vi "適應性控制_線上學習_V7(實際控制).vi"() -> ()   [LabVIEW 2010]
uses:
  <vilib>/DAQmx/read.llb/DAQmx Read (Analog 1D Wfm NChan NSamp).vi
  <vilib>/DAQmx/write.llb/DAQmx Write (Analog DBL 1Chan 1Samp).vi
  <vilib>/DAQmx/create/channels.llb/DAQmx Create Channel (AI-Voltage-Basic).vi
  <vilib>/DAQmx/configure/timing.llb/DAQmx Timing (Sample Clock).vi
  <vilib>/DAQmx/create/channels.llb/DAQmx Create Channel (AO-Voltage-Basic).vi
  <vilib>/daqmx/miscellaneous.llb/DAQmx Fill In Error Info.vi
panel:
  in  "模式選擇":bool=TRUE
  in  "電路 channels":tag="PXI-4472/ai1"
  in  "加速規 channels":tag="PXI-4472/ai0"
  out "輸入訊號":dbl[][](graph)
  out "輸出是否超過範圍":bool
  out "while平均執行時間(ms)":dbl
  out "Time (s)":dbl caption="Elapsed Time (s)"
  in  "error in":errorcluster
  in  "DAQ output":tag="PXI-6733/ao3"
  out "source out":string
  out "當下誤差":dbl=0.1 format="%#_13g"
  out "理想與FIR輸出":dbl[][](graph)
  out "誤差":dbl(graph)
  out "權重(w)":dbl[](array[numeric])
  in  "收斂係數":dbl=0.0001
  in  "order":i32=150
  in  "\"每\"通道取樣頻率":dbl=1000.0 min=1.0 max=10000.0 step=1.0
  in  "stop":bool
  # "版本資訊\nV6:線上學習初版\nV7:設置濾DC固定為1秒\n     新增補償擷取卡取樣與濾波器相位"
  # "ª`·N¨Æ¶µ\n(1)ÂoDC®É­nª`·N¥­§¡¼Æ¾Úªº¸ê®Æ¼Æ,»Ý¬°±±¨î°T¸¹ÀW²vªº¾ã­Ó¶g´Áªº¸ê®Æ¼Æ,¹w³]¥­§¡1¬í¼Æ¾Ú,§Y¥i±±¨î¨ì1Hz°T¸¹\n(2)¦h³q¹D±Ä¼Ë®É,­ì¥»¿é¤Jªº¨ú¼ËÀW²v·|ÀH³q¹D¼Æ¦h¹è³Q¥­§¡±¼,¤H¾÷¤¶­±¬O¿é¤J\"¨C\"³q¹D¨ú¼ËÀW²v"
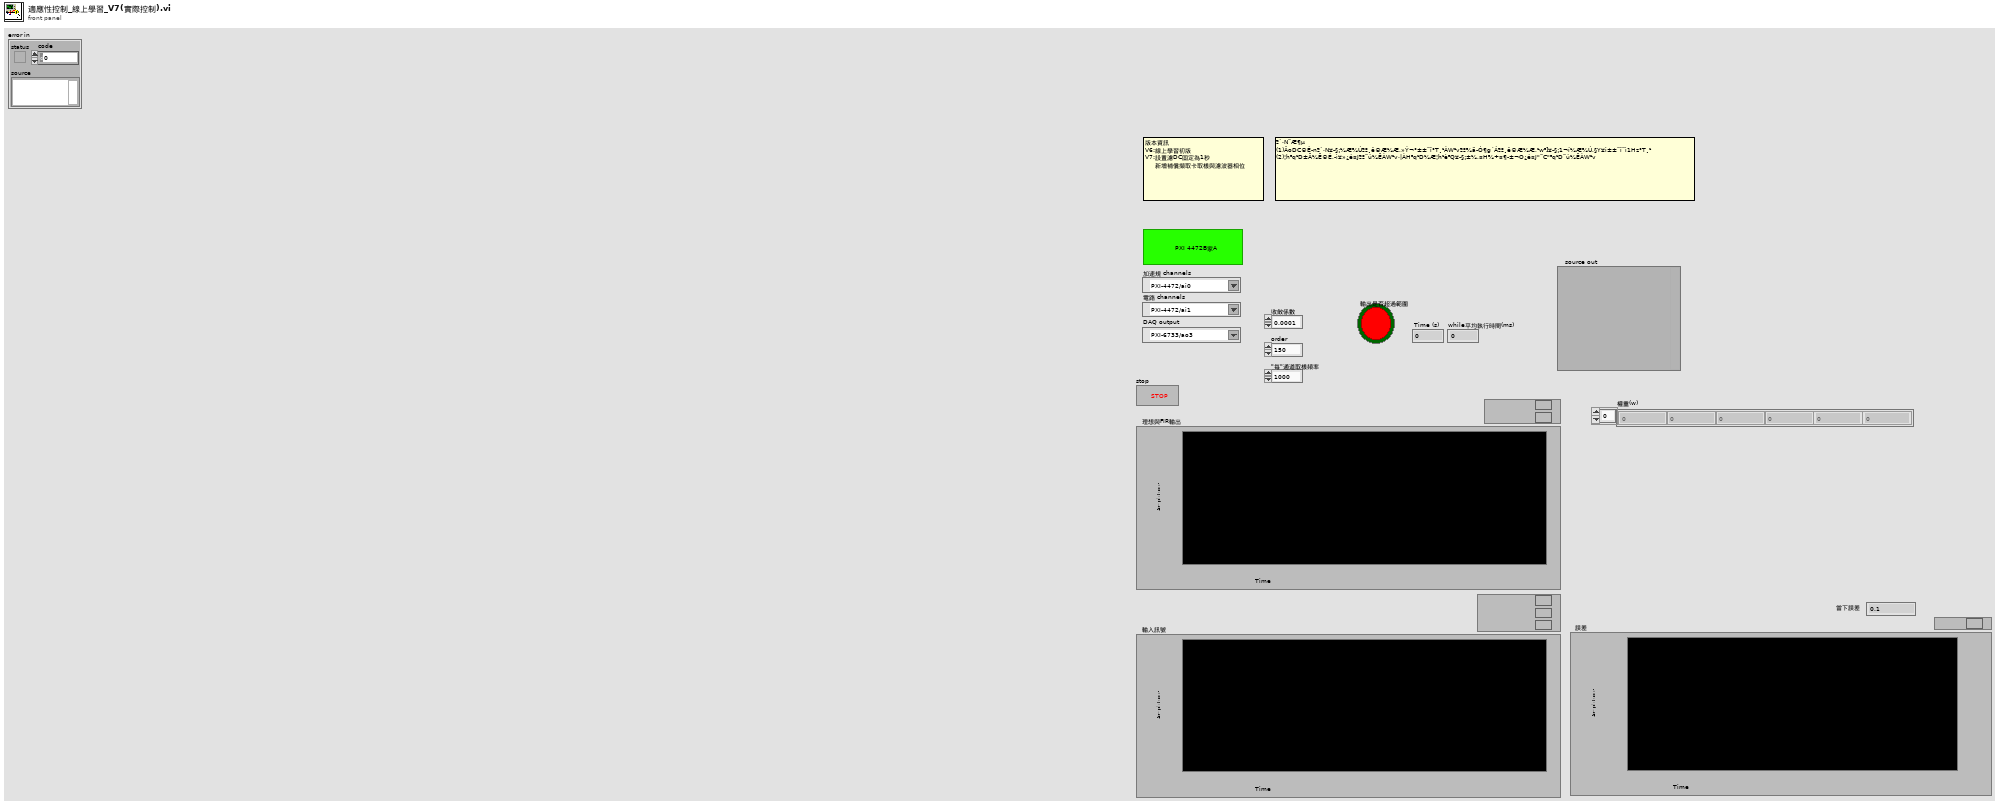
[diagram p1: front panel]
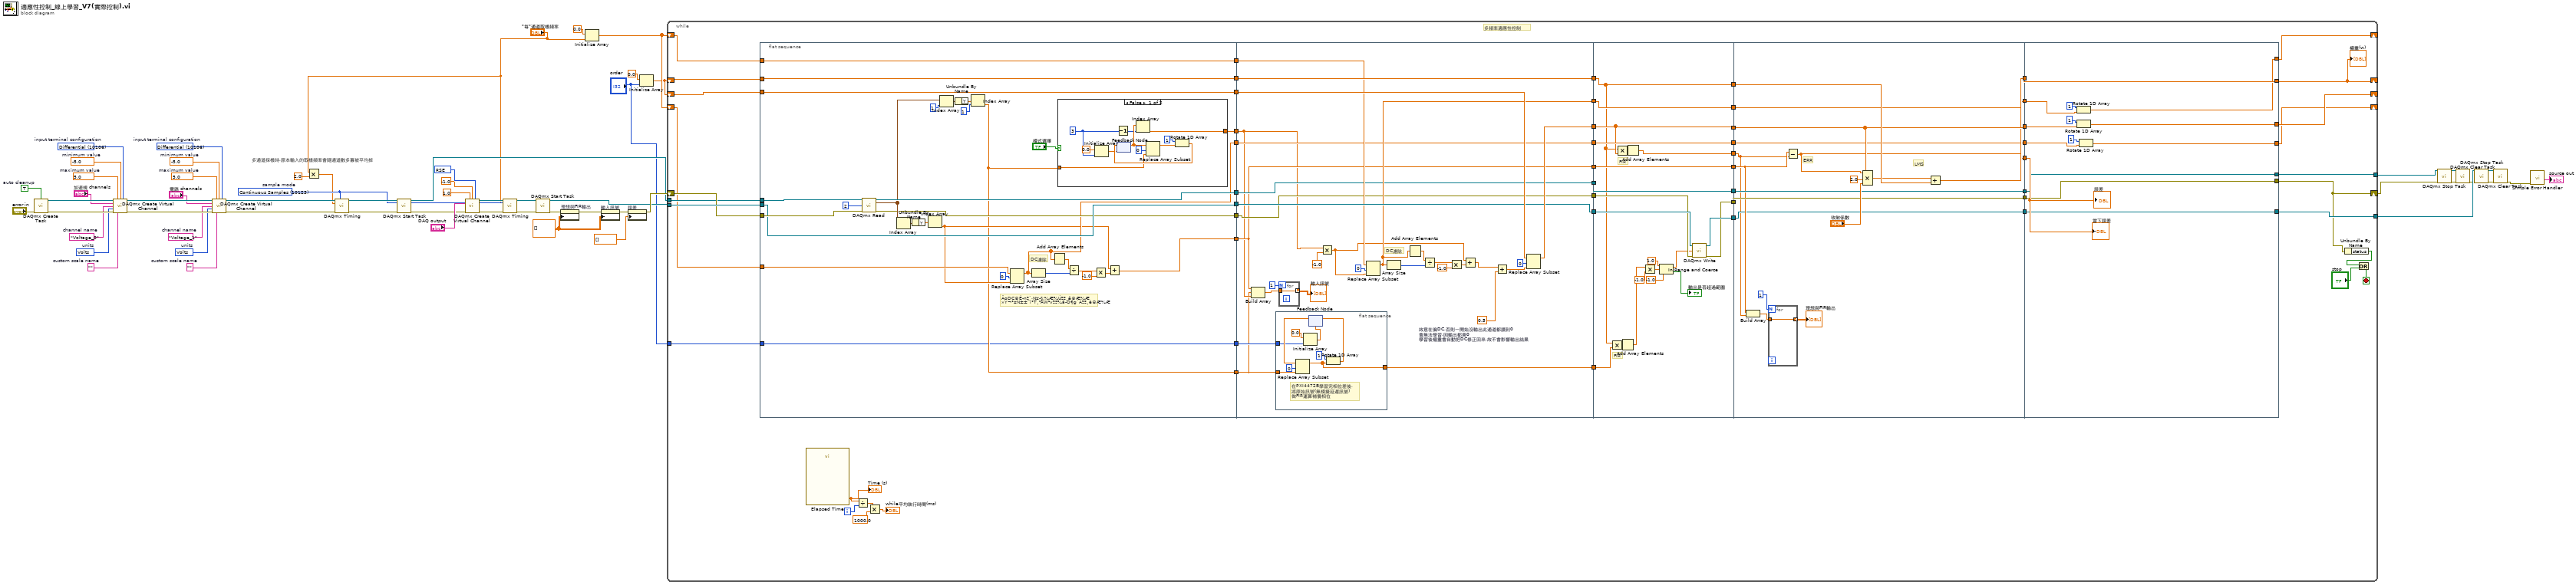
[diagram p0: block diagram]
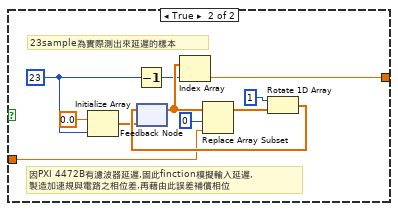
[diagram p2: hidden frame]
diagram:
  w18 = 10123 items=["Finite Samples"=10178, "Continuous Samples"=10123, "Hardware Timed Single Point"=12522]  # sample mode
  w21 = 10106 items=["default"=-1, "RSE"=10083, "NRSE"=10078, "Differential"=10106, "Pseudodifferential"=12529]  # input terminal configuration
  w22 = 10348 items=["Volts"=10348, "From Custom Scale"=10065]  # units
  w23 = "Voltage_1"  # channel name
  w25 = ""  # custom scale name
  w26 = -5.0  # minimum value
  w27 = 5.0  # maximum value
  w28 = 10106 items=["default"=-1, "RSE"=10083, "NRSE"=10078, "Differential"=10106, "Pseudodifferential"=12529]  # input terminal configuration
  w29 = 10348 items=["Volts"=10348, "From Custom Scale"=10065]  # units
  w30 = "Voltage_0"  # channel name
  w32 = ""  # custom scale name
  w33 = -5.0  # minimum value
  w34 = 5.0  # maximum value
  w36 = TRUE  # auto cleanup
  w54 = 10083 items=["Default"=-1, "RSE"=10083, "Differential"=10106, "Pseudodifferential"=12529] ("output terminal configuration")
  w8 = dbl[][] [] ("History Data")
  # "多通道採樣時,原本輸入的取樣頻率會隨通道數多寡被平均掉"
  n1 = call <vilib>:"DAQmx Create Task.vi"("auto cleanup"=w36, "error in"="error in") -> ("task out"=w35:refnum<k21>, "error out"=w37:errorcluster)  [unwired: 12 in]
  n2 = call-poly <vilib>:"DAQmx Create Virtual Channel.vi"("task in"=w35, "maximum value"=w34, "minimum value"=w33, "input terminal configuration"=w28, "physical channels"="加速規 channels", "name to assign"=w30, "units"=w29, "error in"=w37, "custom scale name"=w32) -> ("task out"=w14:refnum<k21>, "error out"=w31:errorcluster)  [unwired: 5 in]
  n3 = call-poly <vilib>:"DAQmx Create Virtual Channel.vi"("task in"=w14, "maximum value"=w27, "minimum value"=w26, "input terminal configuration"=w21, "physical channels"="電路 channels", "name to assign"=w23, "units"=w22, "error in"=w31, "custom scale name"=w25) -> ("task out"=w20:refnum<k21>, "error out"=w24:errorcluster)  [unwired: 5 in]
  n4 = Multiply(x="\"每\"通道取樣頻率", y=2.0) -> (x*y=w5:dbl)
  n5 = call-poly <vilib>:"DAQmx Timing.vi"("task/channels in"=w20, "sample mode"=w18, "rate"=w5, "error in"=w24) -> ("task out"=w19:refnum<k21>, "error out"=w15:errorcluster)  [unwired: 10 in]
  n6 = call <vilib>:"DAQmx Start Task.vi"("task/channels in"=w19, "error in"=w15) -> ("task out"=w16:refnum<k21>, "error out"=w42:errorcluster)  [unwired: 12 in]
  n7 = call-poly <vilib>:"DAQmx Create Virtual Channel.vi"("maximum value"=1.0, "minimum value"=-1.0, "output terminal configuration"=w54, "physical channels"="DAQ output", "error in"=w42) -> ("task out"=w55:refnum<k21>, "error out"=w58:errorcluster)  [unwired: 9 in]
  n8 = call-poly <vilib>:"DAQmx Timing.vi"("task/channels in"=w55, "sample mode"=w18, "rate"="\"每\"通道取樣頻率", "error in"=w58) -> ("task out"=w56:refnum<k21>, "error out"=w57:errorcluster)  [unwired: 10 in]
  n9 = call <vilib>:"DAQmx Start Task.vi"("task/channels in"=w56, "error in"=w57) -> ("task out"=w12:refnum<k21>, "error out"=w17:errorcluster)  [unwired: 12 in]
  n10 = property on="理想與FIR輸出" class="WFChart (strict)"(error in=w17, "History Data"=w8) -> (error out=w10:errorcluster)  [unwired: 1 in, 1 out]
  n11 = Initialize Array(0.0 ("element"), "\"每\"通道取樣頻率") -> (w4:dbl[])
  n12 = property on="輸入訊號" class="WFChart (strict)"(error in=w10, "History Data"=w8) -> (error out=w9:errorcluster)  [unwired: 1 in, 1 out]
  n13 = property on="誤差" class="WFChart (strict)"(error in=w9, "History Data"=dbl[] []) -> (error out=w40:errorcluster)  [unwired: 1 in, 1 out]
  n14 = Initialize Array(0.0 ("element"), "order") -> (w3:dbl[])
  n15 = while {
    shift-right: [w107] -> _
    shift-left: w3 -> [w119]
    shift-right: [w111] -> _
    shift-left: w3 -> [w115]
    tunnel: w12 -> [w106]
    tunnel: [w92] -> w49
    tunnel: [w91] -> w48
    shift-right: [w78] -> _
    shift-left: w4 -> [w88]
    tunnel: w16 -> [w80]
    shift-right: [w79] -> w13
    shift-left: w40 -> [w105]
    shift-right: [w70] -> _
    shift-left: w4 -> [w71]
    tunnel: "order" -> [w61]
    i -> [w65]
    stop <- w89 stop-if-true
    # "多頻率適應性控制"
    n16 = flat-sequence {
      tunnel: [w150] -> w120
      tunnel: w119 -> [w150]
      tunnel: [w149] -> w116
      tunnel: w115 -> [w149]
      tunnel: w106 -> [w137]
      tunnel: w105 -> [w147]
      tunnel: [w146] -> w104
      tunnel: [w136] -> w103
      tunnel: [w137] -> w96
      tunnel: w88 -> [w148]
      tunnel: [w148] -> w87
      tunnel: w80 -> [w139]
      tunnel: [w124] -> w77
      tunnel: [w128] -> w76
      tunnel: w71 -> [w129]
      tunnel: [w127] -> w66
      tunnel: [w123] -> w64
      tunnel: w61 -> [w122]
      tunnel: [w122] -> w62
      tunnel: w120 -> [w199]
      tunnel: [w201] -> w118
      tunnel: [w200] -> w117
      tunnel: w116 -> [w200]
      tunnel: w104 -> [w188]
      tunnel: w103 -> [w187]
      tunnel: [w187] -> w102
      tunnel: [w188] -> w99
      tunnel: [w198] -> w97
      tunnel: w96 -> [w198]
      tunnel: w87 -> [w192]
      tunnel: [w191] -> w86
      tunnel: [w183] -> w81
      tunnel: w77 -> [w174]
      tunnel: w76 -> [w183]
      tunnel: [w182] -> w67
      tunnel: w66 -> [w182]
      tunnel: w64 -> [w173]
      tunnel: [w176] -> w63
      tunnel: w62 -> [w175]
      tunnel: w118 -> [w217]
      tunnel: w117 -> [w213]
      tunnel: [w213] -> w114
      tunnel: [w216] -> w113
      tunnel: [w217] -> w112
      tunnel: w102 -> [w220]
      tunnel: [w219] -> w101
      tunnel: w99 -> [w231]
      tunnel: [w231] -> w98
      tunnel: w97 -> [w224]
      tunnel: [w223] -> w95
      tunnel: w86 -> [w230]
      tunnel: [w230] -> w85
      tunnel: [w229] -> w82
      tunnel: w81 -> [w229]
      tunnel: [w222] -> w68
      tunnel: w67 -> [w222]
      tunnel: w63 -> [w214]
      tunnel: w114 -> [w249]
      tunnel: w113 -> [w233]
      tunnel: w112 -> [w245]
      tunnel: [w243] -> w110
      tunnel: [w245] -> w109
      tunnel: [w237] -> w108
      tunnel: w101 -> [w242]
      tunnel: [w242] -> w100
      tunnel: w98 -> [w241]
      tunnel: w95 -> [w236]
      tunnel: [w236] -> w94
      tunnel: [w241] -> w93
      tunnel: w85 -> [w240]
      tunnel: [w240] -> w84
      tunnel: w82 -> [w238]
      tunnel: [w234] -> w69
      tunnel: w68 -> [w234]
      tunnel: [w264] -> w111
      tunnel: w110 -> [w264]
      tunnel: w109 -> [w261]
      tunnel: [w263] -> w107
      tunnel: w108 -> [w260]
      tunnel: w100 -> [w259]
      tunnel: [w259] -> w79
      tunnel: w94 -> [w257]
      tunnel: w93 -> [w258]
      tunnel: [w258] -> w92
      tunnel: [w257] -> w91
      tunnel: [w254] -> w78
      tunnel: w84 -> [w255]
      tunnel: [w252] -> w70
      tunnel: w69 -> [w251]
      frame #0 {
        # "ÂoDC®É­nª`·N¥­§¡¼Æ¾Úªº¸ê®Æ¼Æ\n»Ý¬°¥N±±¨î°T¸¹ÀW²vªº¾ã­Ó¶g´Áªº¸ê®Æ¼Æ"
        # "DC濾除"
        n17 = call-poly <vilib>:"DAQmx Read.vi"("task/channels in"=w139, "number of samples per channel"=2, "error in"=w147) -> ("task out"=w146:refnum<k21>, "data"=w140:waveform(dbl)[], "error out"=w136:errorcluster)  [unwired: 10 in]
        n18 = Index Array(array=w140) -> (element=w145:waveform(dbl))  [unwired: 1 in]
        n19 = Unbundle By Name(w145) -> ("Y"=w144:dbl[])
        n20 = Index Array(array=w144) -> (element=w126:dbl)  [unwired: 1 in]
        n21 = Index Array(array=w140, index=1) -> (element=w143:waveform(dbl))
        n22 = Unbundle By Name(w143) -> ("Y"=w142:dbl[])
        n23 = Index Array(array=w142, index=1) -> (element=w123:dbl)
        n24 = Replace Array Subset(array=w129, new element=w126, index=0) -> (w127:dbl[])
        n25 = Array Size(array=w127) -> (size(s)=w133:i32)
        n26 = Add Array Elements(numeric array=w127) -> (sum=w132:dbl)
        n27 = case shown="False" "模式選擇" {
          tunnel: [w151 w169] -> w124
          tunnel: w123 -> [w152 w166]
          frame False {
            w153 = 3 ("index")
            n28 = Initialize Array(0.0 ("element"), w153) -> (w155:dbl[])
            n29 = Decrement(x=w153) -> (x-1=w154:i32)
            n30 = feedback #1(w155) -> (w157:dbl[])
            n31 = Index Array(array=w157, index=w154) -> (element=w151:dbl)
            n32 = Replace Array Subset(array=w157, new element=w152, index=0) -> (w160:dbl[])
            n33 = Rotate 1D Array(1:w160, 2:1 ("n")) -> (0:w158:dbl[])
            n34 = feedback-in #1(w158) -> ()
          }
          frame True {
            w162 = 23 ("index")
            # "23sample為實際測出來延遲的樣本"
            # "因PXI 4472B有濾波器延遲,固此finction模擬輸入延遲,\n製造加速規與電路之相位差,再藉由此誤差補償相位"
            n35 = Initialize Array(0.0 ("element"), w162) -> (w164:dbl[])
            n36 = Decrement(x=w162) -> (x-1=w163:i32)
            n37 = feedback #2(w164) -> (w167:dbl[])
            n38 = Index Array(array=w167, index=w163) -> (element=w169:dbl)
            n39 = Replace Array Subset(array=w167, new element=w166, index=0) -> (w171:dbl[])
            n40 = Rotate 1D Array(1:w171, 2:1 ("n")) -> (0:w168:dbl[])
            n41 = feedback-in #2(w168) -> ()
          }
        }
        n42 = Divide(x=w132, y=w133) -> (x/y=w134:dbl)
        n43 = Multiply(x=w134, y=-1.0) -> (x*y=w135:dbl)
        n44 = Add(x=w126, y=w135) -> (x+y=w128:dbl)
      }
      frame #1 {
        w180 = 0.5  # 故意在偏DC,否則一開始沒輸出此通道都讀到0 會無法學習,因輸出都乘0 學習後權重會自動把DC修正回來,故不會影響輸出結果
        # "DC濾除"
        n45 = Build Array(w183, w173, w174) -> (w185:dbl[])
        n46 = flat-sequence {
          tunnel: w173 -> [w209]
          tunnel: [w203] -> w176
          tunnel: w175 -> [w202]
          frame #0 {
            # "在PXI4472B學習完相位差後,\n將原始訊號(無模擬延遲訊號)\n做FIR運算補償相位"
            n47 = Initialize Array(0.0 ("element"), w202) -> (w205:dbl[])
            n48 = feedback #3(w205) -> (w207:dbl[])
            n49 = Replace Array Subset(array=w207, new element=w209, index=0) -> (w203:dbl[])
            n50 = Rotate 1D Array(1:w203, 2:1 ("n")) -> (0:w208:dbl[])
            n51 = feedback-in #3(w208) -> ()
          }
        }
        n52 = for {
          N: 1 -> [_]
          tunnel: w185 -> [w211]
          tunnel: [w211] -> w179 mode=indexing
        }
        "輸入訊號" <- w179
        n53 = Multiply(x=w174, y=-1.0) -> (x*y=w186:dbl)
        n54 = Replace Array Subset(array=w192, new element=w186, index=0) -> (w191:dbl[])
        n55 = Array Size(array=w191) -> (size(s)=w195:i32)
        n56 = Add Array Elements(numeric array=w191) -> (sum=w194:dbl)
        n57 = Divide(x=w194, y=w195) -> (x/y=w196:dbl)
        n58 = Multiply(x=w196, y=-1.0) -> (x*y=w197:dbl)
        n59 = Add(x=w186, y=w197) -> (x+y=w181:dbl)
        n60 = Add(x=w181, y=w180) -> (x+y=w178:dbl)
        n61 = Replace Array Subset(array=w199, new element=w178, index=0) -> (w201:dbl[])
      }
      frame #2 {
        # "FIR"
        # "FIR"
        n62 = Multiply(x=w213, y=w214) -> (x*y=w215:dbl[])
        n63 = Multiply(x=w213, y=w217) -> (x*y=w232:dbl[])
        n64 = Add Array Elements(numeric array=w215) -> (sum=w212:dbl)
        n65 = Add Array Elements(numeric array=w232) -> (sum=w216:dbl)
        n66 = Multiply(x=w212, y=-1.0) -> (x*y=w227:dbl)
        n67 = In Range and Coerce(upper limit=1.0, x=w227, lower limit=-1.0 ("upper limit")) -> (coerced(x)=w218:dbl, In Range?=→"輸出是否超過範圍":bool)
        n68 = call-poly <vilib>:"DAQmx Write.vi"("task/channels in"=w224, "data"=w218, "error in"=w220) -> ("task out"=w223:refnum<k21>, "error out"=w219:errorcluster)  [unwired: 10 in, 1 out]
      }
      frame #3 {
        # "LMS"
        # "ERR"
        n69 = Build Array(w238, w233) -> (w248:dbl[])
        n70 = for {
          N: 1 -> [_]
          tunnel: [w250] -> w235 mode=indexing
          tunnel: w248 -> [w250]
        }
        "理想與FIR輸出" <- w235
        n71 = Subtract(x=w238, y=w233) -> (x-y=w237:dbl)
        n72 = Compound Arithmetic op=MULTIPLY(w237, w245, 2.0, "收斂係數") -> (w244:dbl[])
        n73 = Add(x=w244, y=w249) -> (x+y=w243:dbl[])
      }
      frame #4 {
        n74 = Rotate 1D Array(1:w255, 2:1 ("n")) -> (0:w254:dbl[])
        n75 = Rotate 1D Array(1:w261, 2:1 ("n")) -> (0:w263:dbl[])
        n76 = Rotate 1D Array(1:w251, 2:1 ("n")) -> (0:w252:dbl[])
        "誤差" <- w260
        "當下誤差" <- w260
      }
    }
    n77 = call "Elapsed Time"() -> ("Elapsed Time (s)"=w75:dbl)  [unwired: 12 in, 7 out]
    "Time (s)" <- w75
    n78 = Divide(x=w75, y=w65) -> (x/y=w74:dbl)
    n79 = Multiply(x=w74, y=1000.0) -> (x*y=→"while平均執行時間(ms)":dbl)
    n80 = Unbundle By Name(w79) -> ("status"=w83:bool)
    n81 = Or(x=w83, y="stop") -> (x .or. y?=w89:bool)
    "權重(w)" <- w111
  }
  n82 = call <vilib>:"DAQmx Stop Task.vi"("task/channels in"=w49, "error in"=w13) -> ("task out"=w51:refnum<k21>, "error out"=w50:errorcluster)  [unwired: 12 in]
  n83 = call <vilib>:"DAQmx Clear Task.vi"("task in"=w51, "error in"=w50) -> ("error out"=w41:errorcluster)  [unwired: 13 in]
  n84 = call <vilib>:"DAQmx Stop Task.vi"("task/channels in"=w48, "error in"=w41) -> ("task out"=w46:refnum<k21>, "error out"=w47:errorcluster)  [unwired: 12 in]
  n85 = call <vilib>:"DAQmx Clear Task.vi"("task in"=w46, "error in"=w47) -> ("error out"=w39:errorcluster)  [unwired: 13 in]
  n86 = call <vilib>:"Simple Error Handler.vi"("error in (no error)"=w39) -> ("source out"=→"source out":string)  [unwired: 4 in, 4 out]
